vi "Cockpit UDP Receiver IRISSv2.vi"(8 "error in":errorcluster, 11 "port":refnum<k16>) -> (0 "deltaRoll":sgl, 1 "deltaZ":sgl, 2 "deltaY":sgl, 3 "deltaX":sgl, 4 "gripper":sgl)   [LabVIEW 2016]
panel:
  out "error out":errorcluster
  out "connection ID out":refnum<k16>
  in  "stop 2":bool
  out "deltaX 2":sgl
  out "data out 2":string
  out "length 2":i32
  out "deltaY 2":sgl
  out "deltaZ 2":sgl
  out "deltaRoll 2":sgl
  out "gripper 2":sgl
  out "down_pedal 2":sgl format="%.2f"
  out "up_pedal 2":bool
  out "left_pedal 2":bool
  out "right_pedal 2":bool
  out "Waveform Chart 8":sgl(graph)
  out "Waveform Chart 7":sgl(graph)
  out "Waveform Chart 6":sgl(graph)
  out "Waveform Chart 5":sgl(graph)
  out "Waveform Chart 4":sgl(graph)
  out "Waveform Chart 3":sgl(graph)
  out "Waveform Chart 2":sgl(graph)
  out "Waveform Chart":sgl(graph)
  out "right_pedal":bool
  out "left_pedal":bool
  out "up_pedal":bool
  out "down_pedal":sgl format="%.2f"
  out "length":i32
  out "data out":string
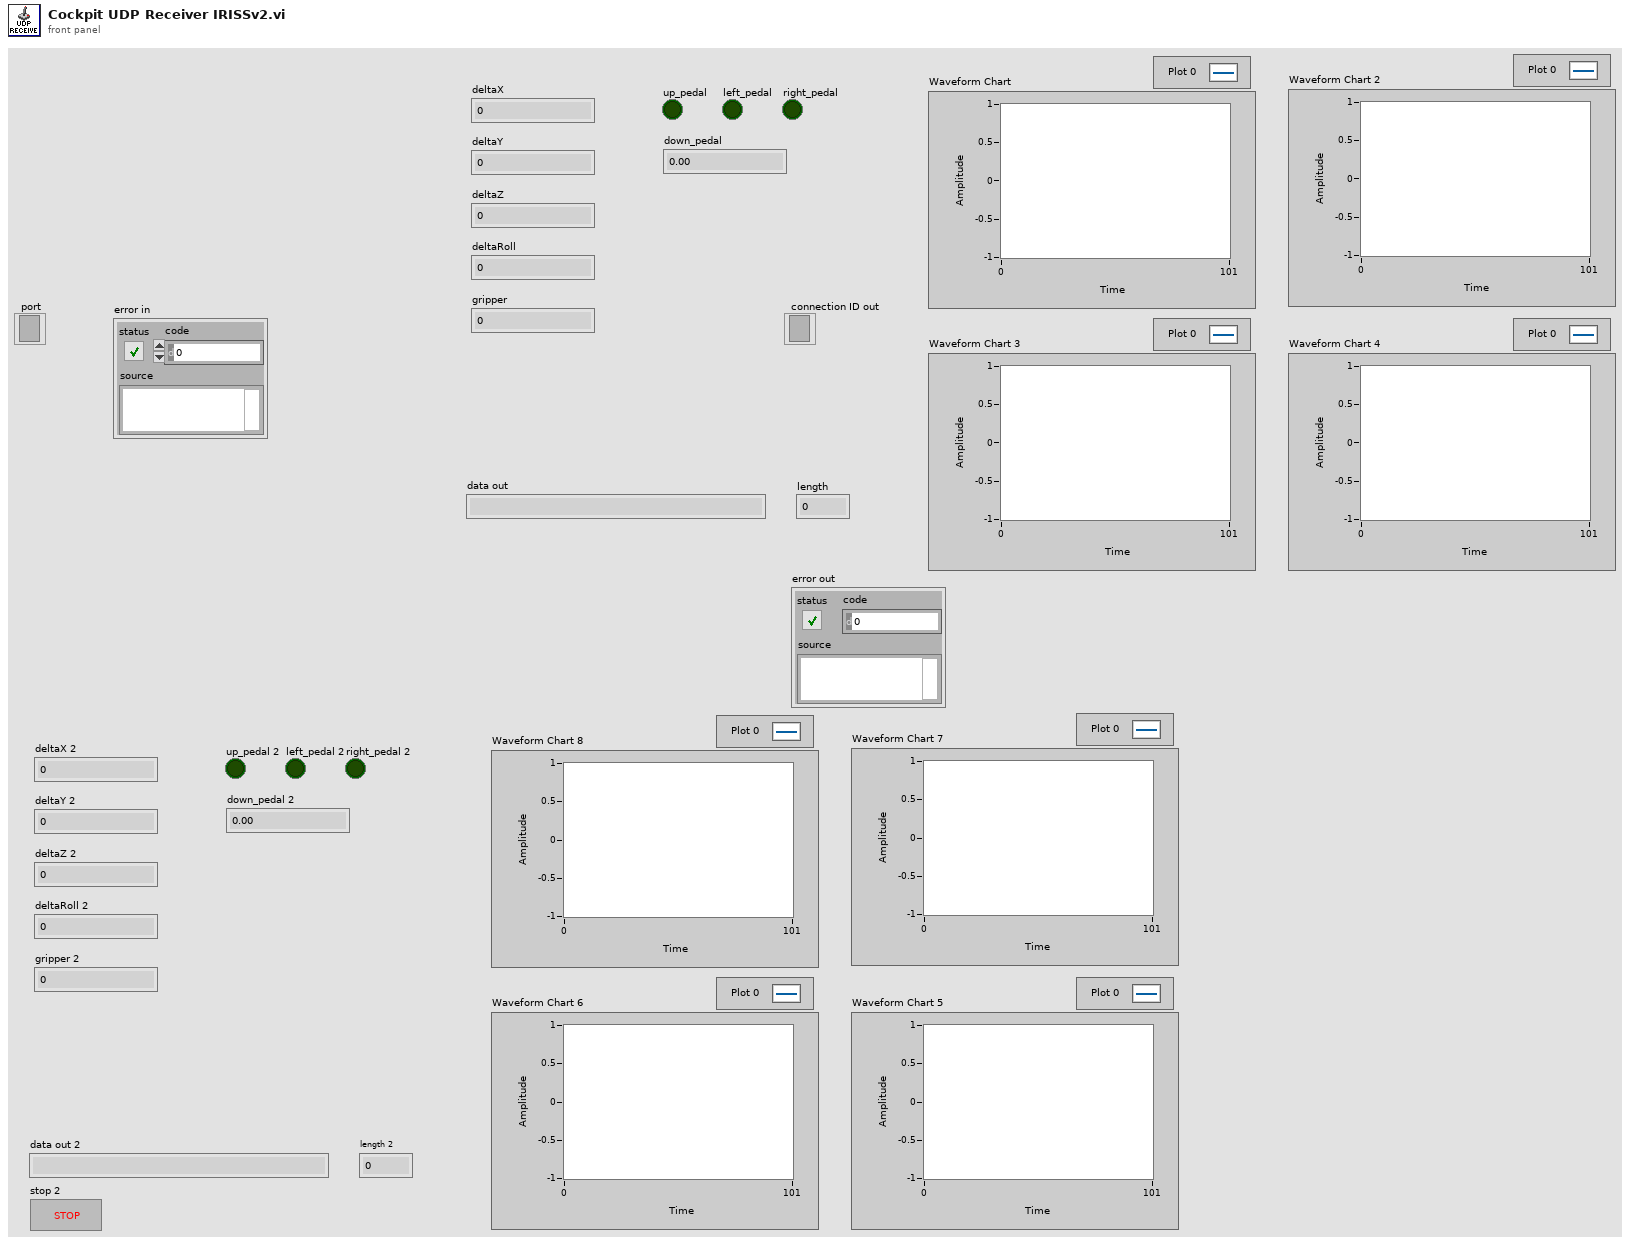
[diagram p1: front panel]
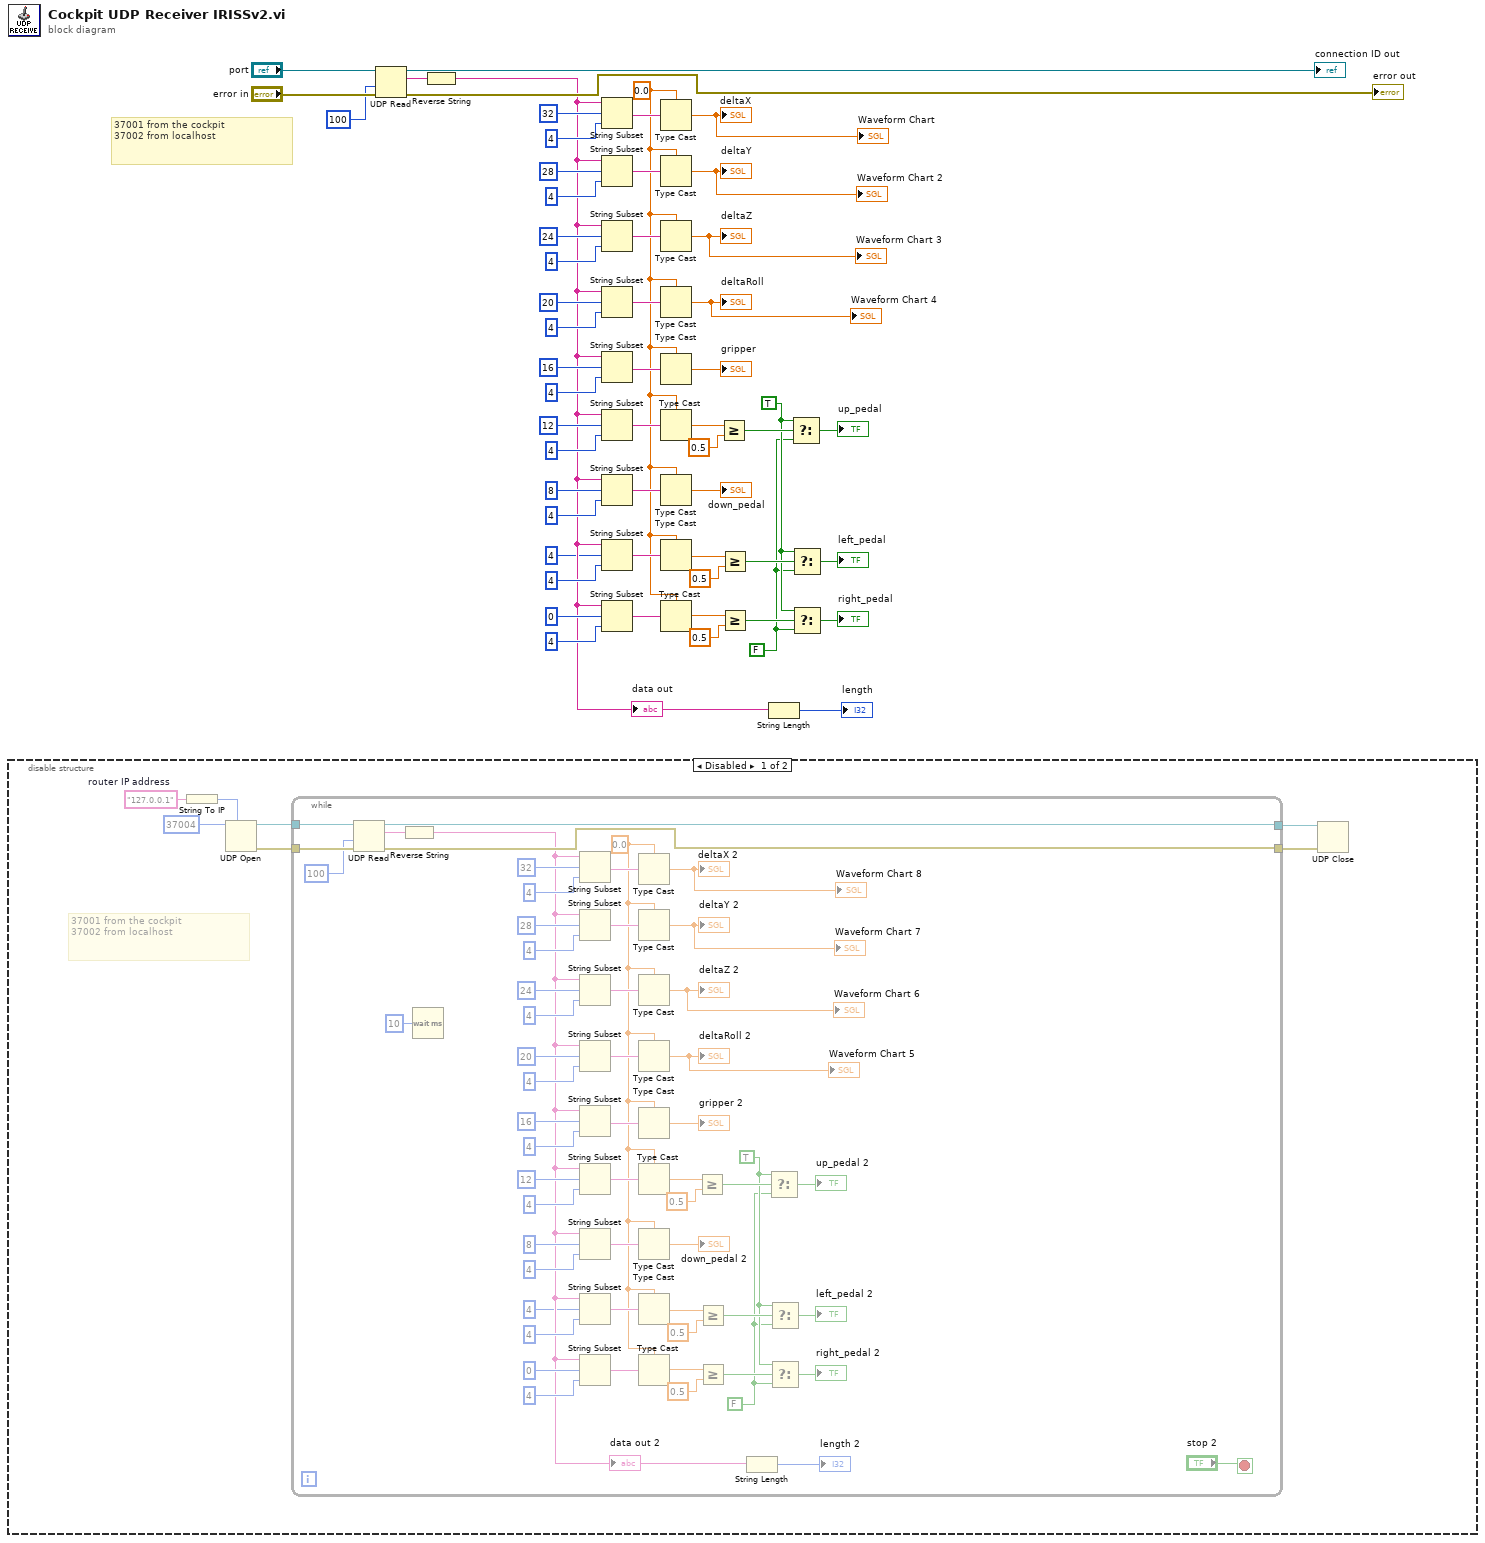
[diagram p0: block diagram]
diagram:
  w10 = FALSE
  w11 = TRUE
  w21 = sgl 0.0
  # "37001 from the cockpit\n37002 from localhost"
  n1 = disable-structure shown="Disabled" {
    frame Disabled {
      w58 = "127.0.0.1"  # router IP address
      # "37001 from the cockpit\n37002 from localhost"
      n2 = String To IP(1:w58) -> (0:w57:u32)
      n3 = UDP Open(7:w57, 11:u16 37004 ("port")) -> (port=w62:refnum<k16>, 0:w60:errorcluster)  [unwired: 3 in, 1 out]
      n4 = while {
        tunnel: w62 -> [w121]
        tunnel: [w119] -> w61
        tunnel: w60 -> [w90]
        tunnel: [w89] -> w59
        stop <- "stop 2" stop-if-true
        w74 = FALSE
        w75 = TRUE
        w85 = sgl 0.0
        n5 = UDP Read(connection ID=w121, timeout ms (25000)=100, 8:w90) -> (data out=w88:string, error out=w89:errorcluster, 3:w119:refnum<k16>)  [unwired: 1 in, 2 out]
        n6 = Reverse String(1:w88) -> (0:w87:string)
        "data out 2" <- w87
        n7 = Wait (ms)(milliseconds to wait=u32 10) -> ()  [unwired: 1 out]
        n8 = String Subset(string=w87, offset (0)=32, length (rest)=4 ("offset (0)")) -> (substring=w116:string)
        n9 = String Subset(string=w87, offset (0)=28, length (rest)=4 ("offset (0)")) -> (substring=w108:string)
        n10 = String Subset(string=w87, offset (0)=24, length (rest)=4 ("offset (0)")) -> (substring=w107:string)
        n11 = String Subset(string=w87, offset (0)=20, length (rest)=4 ("offset (0)")) -> (substring=w106:string)
        n12 = String Subset(string=w87, offset (0)=16, length (rest)=4 ("offset (0)")) -> (substring=w96:string)
        n13 = String Subset(string=w87, offset (0)=12, length (rest)=4 ("offset (0)")) -> (substring=w103:string)
        n14 = String Subset(string=w87, offset (0)=8, length (rest)=4 ("offset (0)")) -> (substring=w104:string)
        n15 = String Subset(string=w87, offset (0)=4, length (rest)=4 ("offset (0)")) -> (substring=w105:string)
        n16 = String Subset(string=w87, offset (0)=0, length (rest)=4 ("offset (0)")) -> (substring=w91:string)
        n17 = Type Cast(type=w85, x=w116) -> (*(type *) &x=→"deltaX 2" →"Waveform Chart 8":sgl)
        n18 = Type Cast(type=w85, x=w108) -> (*(type *) &x=→"deltaY 2" →"Waveform Chart 7":sgl)
        n19 = Type Cast(type=w85, x=w107) -> (*(type *) &x=→"deltaZ 2" →"Waveform Chart 6":sgl)
        n20 = Type Cast(type=w85, x=w106) -> (*(type *) &x=→"deltaRoll 2" →"Waveform Chart 5":sgl)
        n21 = Type Cast(type=w85, x=w96) -> (*(type *) &x=→"gripper 2":sgl)
        n22 = Type Cast(type=w85, x=w103) -> (*(type *) &x=w82:sgl)
        n23 = Type Cast(type=w85, x=w104) -> (*(type *) &x=→"down_pedal 2":sgl)
        n24 = Type Cast(type=w85, x=w105) -> (*(type *) &x=w76:sgl)
        n25 = Type Cast(type=w85, x=w91) -> (*(type *) &x=w77:sgl)
        n26 = Greater Or Equal?(x=w82, y=sgl 0.5) -> (x >= y?=w84:bool)
        n27 = Greater Or Equal?(x=w76, y=sgl 0.5) -> (x >= y?=w80:bool)
        n28 = Greater Or Equal?(x=w77, y=sgl 0.5) -> (x >= y?=w79:bool)
        n29 = String Length(string=w87) -> (length=→"length 2":i32)
        n30 = Select(t=w75, s=w84, f=w74) -> (s? t:f=→"up_pedal 2":bool)
        n31 = Select(t=w75, s=w80, f=w74) -> (s? t:f=→"left_pedal 2":bool)
        n32 = Select(t=w75, s=w79, f=w74) -> (s? t:f=→"right_pedal 2":bool)
      }
      n33 = UDP Close(connection ID=w61, 8:w59) -> ()  [unwired: 2 out]
    }
    frame Enabled {
    }
  }
  n34 = UDP Read(connection ID="port", timeout ms (25000)=100, 8:"error in") -> (data out=w24:string, error out=→"error out":errorcluster, 3:→"connection ID out":refnum<k16>)  [unwired: 1 in, 2 out]
  n35 = Reverse String(1:w24) -> (0:w23:string)
  "data out" <- w23
  n36 = String Subset(string=w23, offset (0)=32, length (rest)=4 ("offset (0)")) -> (substring=w50:string)
  n37 = String Subset(string=w23, offset (0)=28, length (rest)=4 ("offset (0)")) -> (substring=w42:string)
  n38 = String Subset(string=w23, offset (0)=24, length (rest)=4 ("offset (0)")) -> (substring=w41:string)
  n39 = String Subset(string=w23, offset (0)=20, length (rest)=4 ("offset (0)")) -> (substring=w40:string)
  n40 = String Subset(string=w23, offset (0)=16, length (rest)=4 ("offset (0)")) -> (substring=w30:string)
  n41 = String Subset(string=w23, offset (0)=12, length (rest)=4 ("offset (0)")) -> (substring=w37:string)
  n42 = String Subset(string=w23, offset (0)=8, length (rest)=4 ("offset (0)")) -> (substring=w38:string)
  n43 = String Subset(string=w23, offset (0)=4, length (rest)=4 ("offset (0)")) -> (substring=w39:string)
  n44 = String Subset(string=w23, offset (0)=0, length (rest)=4 ("offset (0)")) -> (substring=w25:string)
  n45 = Type Cast(type=w21, x=w50) -> (*(type *) &x=→"deltaX" →"Waveform Chart":sgl)
  n46 = Type Cast(type=w21, x=w42) -> (*(type *) &x=→"deltaY" →"Waveform Chart 2":sgl)
  n47 = Type Cast(type=w21, x=w41) -> (*(type *) &x=→"deltaZ" →"Waveform Chart 3":sgl)
  n48 = Type Cast(type=w21, x=w40) -> (*(type *) &x=→"deltaRoll" →"Waveform Chart 4":sgl)
  n49 = Type Cast(type=w21, x=w30) -> (*(type *) &x=→"gripper":sgl)
  n50 = Type Cast(type=w21, x=w37) -> (*(type *) &x=w18:sgl)
  n51 = Type Cast(type=w21, x=w38) -> (*(type *) &x=→"down_pedal":sgl)
  n52 = Type Cast(type=w21, x=w39) -> (*(type *) &x=w12:sgl)
  n53 = Type Cast(type=w21, x=w25) -> (*(type *) &x=w13:sgl)
  n54 = Greater Or Equal?(x=w18, y=sgl 0.5) -> (x >= y?=w20:bool)
  n55 = Greater Or Equal?(x=w12, y=sgl 0.5) -> (x >= y?=w16:bool)
  n56 = Greater Or Equal?(x=w13, y=sgl 0.5) -> (x >= y?=w15:bool)
  n57 = String Length(string=w23) -> (length=→"length":i32)
  n58 = Select(t=w11, s=w20, f=w10) -> (s? t:f=→"up_pedal":bool)
  n59 = Select(t=w11, s=w16, f=w10) -> (s? t:f=→"left_pedal":bool)
  n60 = Select(t=w11, s=w15, f=w10) -> (s? t:f=→"right_pedal":bool)
